vi "Action Placeholder.vi"(8 "error in (no error)":errorcluster, 10 "Placeholder":bool, 11 "Actor In":refnum<class "Template.lvclass">) -> (0 "error out":errorcluster, 3 "Actor Out":refnum<class "Template.lvclass">)   [LabVIEW 2020]
uses:
  Artifex Template/Template/Template.lvclass
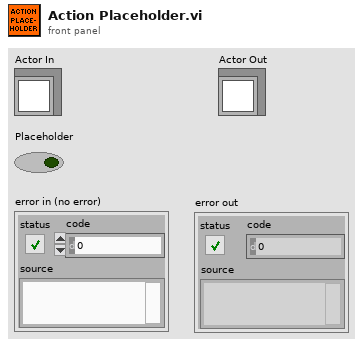
[diagram p1: front panel]
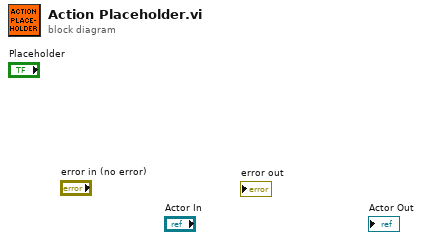
[diagram p0: block diagram]
diagram:
